vi "MCS_Stop All Actions.vi"() -> ()   [LabVIEW 2010]
panel:
  out "error out":errorcluster
  in  "error in (no error)":errorcluster
  in  "MCS System Locator":string
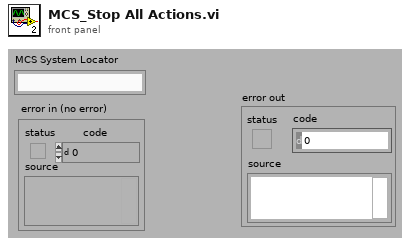
[diagram p1: front panel]
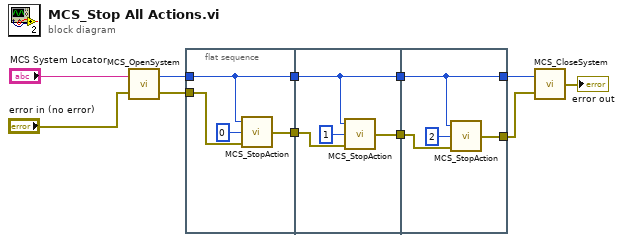
[diagram p0: block diagram]
diagram:
  n1 = call "MCS_OpenSystem.vi"("error in (no error)"="error in (no error)", "MCS System Locator"="MCS System Locator") -> ("error out"=w8:errorcluster, "System Index Out"=w9:u32)
  n2 = flat-sequence {
    tunnel: w9 -> [w15]
    tunnel: w8 -> [w13]
    tunnel: [w15] -> w7
    tunnel: [w12] -> w6
    tunnel: w7 -> [w17]
    tunnel: w6 -> [w18]
    tunnel: [w17] -> w5
    tunnel: [w16] -> w4
    tunnel: [w21] -> w3
    tunnel: w5 -> [w21]
    tunnel: w4 -> [w22]
    tunnel: [w20] -> w2
    frame #0 {
      n3 = call "MCS_StopAction.vi"("error in (no error)"=w13, "Channel Index In"=u32 0, "System Index In"=w15) -> ("error out"=w12:errorcluster)
    }
    frame #1 {
      n4 = call "MCS_StopAction.vi"("error in (no error)"=w18, "Channel Index In"=u32 1, "System Index In"=w17) -> ("error out"=w16:errorcluster)
    }
    frame #2 {
      n5 = call "MCS_StopAction.vi"("error in (no error)"=w22, "Channel Index In"=u32 2, "System Index In"=w21) -> ("error out"=w20:errorcluster)
    }
  }
  n6 = call "MCS_CloseSystem.vi"("error in (no error)"=w2, "System Index In"=w3) -> ("error out"=→"error out":errorcluster)
